vi "Default String File--constant.vi"() -> (3 "Default String File":path)   [LabVIEW 2025]
doc: "This constant defines the default file output for the generated strings."
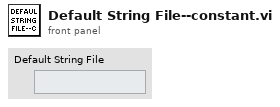
[diagram p1: front panel]
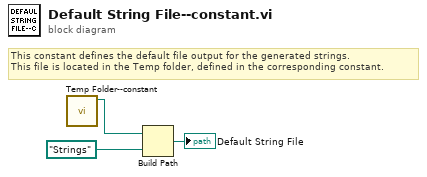
[diagram p0: block diagram]
diagram:
  # "This constant defines the default file output for the generated strings.\nThis file is located in the Temp folder, defined in the corresponding constant."
  n1 = call "Temp Folder--constant.vi"() -> ("Temp Folder"=w1:path)  [unwired: 7 in]
  n2 = Build Path(base path=w1, name or relative path=path "Strings" ("Test Folder")) -> (appended path=→"Default String File":path)
